vi "Auto Repeated.vi"   [LabVIEW 2014]
uses:
  Robot Global Data.vi
types:
  T1 = cluster{"Lifter Down":bool, "Right Infeed":enum16{"Off", "Forward", "Reverse"}, "Left Infeed":enum16{"Off", "Forward", "Reverse"}}
  T2 = typedef "Rendezvous RefNum" = refnum<k1>
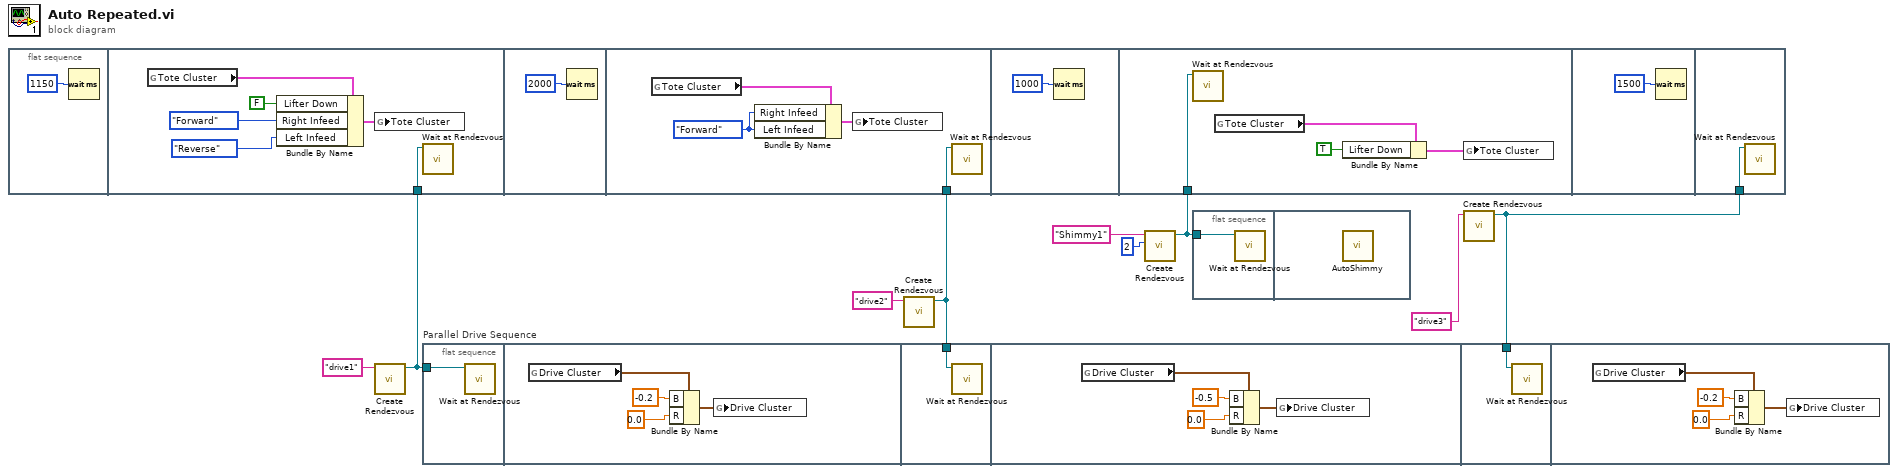
[diagram p0: block diagram]
diagram:
  n1 = flat-sequence {
    tunnel: w8 -> [w11]
    tunnel: w5 -> [w18]
    tunnel: w1 -> [w23]
    tunnel: w4 -> [w28]
    frame #0 {
      n2 = Wait (ms)(milliseconds to wait=u32 1150 ("millisecond multiple")) -> ()  [unwired: 1 out]
    }
    frame #1 {
      n3 = global read "Robot Global Data.vi" "Tote Cluster"() -> (w14:T1)
      n4 = Bundle By Name(cluster=w14, "Lifter Down"=FALSE ("Lifter"), "Right Infeed"=enum16{"Off", "Forward", "Reverse"}."Forward", "Left Infeed"=enum16{"Off", "Forward", "Reverse"}."Reverse") -> (w13:T1)
      n5 = global write "Robot Global Data.vi" "Tote Cluster"(w13) -> ()
      n6 = call <vilib>:"Wait at Rendezvous.vi"("rendezvous"=w11) -> ()  [unwired: 4 in, 3 out]
    }
    frame #2 {
      n7 = Wait (ms)(milliseconds to wait=u32 2000 ("millisecond multiple")) -> ()  [unwired: 1 out]
    }
    frame #3 {
      w19 = enum16{"Off", "Forward", "Reverse"}."Forward" ("Right Infeed")
      n8 = global read "Robot Global Data.vi" "Tote Cluster"() -> (w20:T1)
      n9 = Bundle By Name(cluster=w20, "Right Infeed"=w19, "Left Infeed"=w19) -> (w21:T1)
      n10 = global write "Robot Global Data.vi" "Tote Cluster"(w21) -> ()
      n11 = call <vilib>:"Wait at Rendezvous.vi"("rendezvous"=w18) -> ()  [unwired: 4 in, 3 out]
    }
    frame #4 {
      n12 = Wait (ms)(milliseconds to wait=u32 1000 ("millisecond multiple")) -> ()  [unwired: 1 out]
    }
    frame #5 {
      n13 = call <vilib>:"Wait at Rendezvous.vi"("rendezvous"=w23) -> ()  [unwired: 4 in, 3 out]
      n14 = global read "Robot Global Data.vi" "Tote Cluster"() -> (w25:T1)
      n15 = Bundle By Name(cluster=w25, "Lifter Down"=TRUE ("Lifter")) -> (w24:T1)
      n16 = global write "Robot Global Data.vi" "Tote Cluster"(w24) -> ()
    }
    frame #6 {
      n17 = Wait (ms)(milliseconds to wait=u32 1500 ("millisecond multiple")) -> ()  [unwired: 1 out]
    }
    frame #7 {
      n18 = call <vilib>:"Wait at Rendezvous.vi"("rendezvous"=w28) -> ()  [unwired: 4 in, 3 out]
    }
  }
  n19 = call <vilib>:"Create Rendezvous.vi"("name (unnamed)"="drive1") -> ("rendezvous"=w8:T2)  [unwired: 4 in, 2 out]
  n20 = flat-sequence "Parallel Drive Sequence" {
    tunnel: w8 -> [w29]
    tunnel: w5 -> [w34]
    tunnel: w4 -> [w39]
    frame #0 {
      n21 = call <vilib>:"Wait at Rendezvous.vi"("rendezvous"=w29) -> ()  [unwired: 4 in, 3 out]
    }
    frame #1 {
      n22 = global read "Robot Global Data.vi" "Drive Cluster"() -> (w31:cluster{"A":dbl, "B":dbl, "R":dbl, "Gyro":dbl})
      n23 = Bundle By Name(cluster=w31, "B"=-0.2, "R"=0.0) -> (w32:cluster{"A":dbl, "B":dbl, "R":dbl, "Gyro":dbl})
      n24 = global write "Robot Global Data.vi" "Drive Cluster"(w32) -> ()
    }
    frame #2 {
      n25 = call <vilib>:"Wait at Rendezvous.vi"("rendezvous"=w34) -> ()  [unwired: 4 in, 3 out]
    }
    frame #3 {
      n26 = global read "Robot Global Data.vi" "Drive Cluster"() -> (w36:cluster{"A":dbl, "B":dbl, "R":dbl, "Gyro":dbl})
      n27 = Bundle By Name(cluster=w36, "B"=-0.5, "R"=0.0) -> (w37:cluster{"A":dbl, "B":dbl, "R":dbl, "Gyro":dbl})
      n28 = global write "Robot Global Data.vi" "Drive Cluster"(w37) -> ()
    }
    frame #4 {
      n29 = call <vilib>:"Wait at Rendezvous.vi"("rendezvous"=w39) -> ()  [unwired: 4 in, 3 out]
    }
    frame #5 {
      n30 = global read "Robot Global Data.vi" "Drive Cluster"() -> (w41:cluster{"A":dbl, "B":dbl, "R":dbl, "Gyro":dbl})
      n31 = Bundle By Name(cluster=w41, "B"=-0.2, "R"=0.0) -> (w42:cluster{"A":dbl, "B":dbl, "R":dbl, "Gyro":dbl})
      n32 = global write "Robot Global Data.vi" "Drive Cluster"(w42) -> ()
    }
  }
  n33 = call <vilib>:"Create Rendezvous.vi"("name (unnamed)"="drive2") -> ("rendezvous"=w5:T2)  [unwired: 4 in, 2 out]
  n34 = call <vilib>:"Create Rendezvous.vi"("size (2)"=2, "name (unnamed)"="Shimmy1") -> ("rendezvous"=w1:T2)  [unwired: 3 in, 2 out]
  n35 = flat-sequence {
    tunnel: w1 -> [w44]
    frame #0 {
      n36 = call <vilib>:"Wait at Rendezvous.vi"("rendezvous"=w44) -> ()  [unwired: 4 in, 3 out]
    }
    frame #1 {
      n37 = call "AutoShimmy.vi"() -> ()  [unwired: 12 in]
    }
  }
  n38 = call <vilib>:"Create Rendezvous.vi"("name (unnamed)"="drive3") -> ("rendezvous"=w4:T2)  [unwired: 4 in, 2 out]
